vi "Get Header.vi"(8 "error in (no error)":errorcluster, 9 "Default":string, 10 "Header":string, 11 "Request in":refnum<class "Request.lvclass">) -> (0 "error out":errorcluster, 1 "Found?":bool, 2 "Value":string, 3 "Request out":refnum<class "Request.lvclass">)   [LabVIEW 2023, in "Request.lvclass"]
doc: "Returns the value for a given header, if it exists."
uses:
  Request.lvclass
  Request.lvclass/Request.ctl
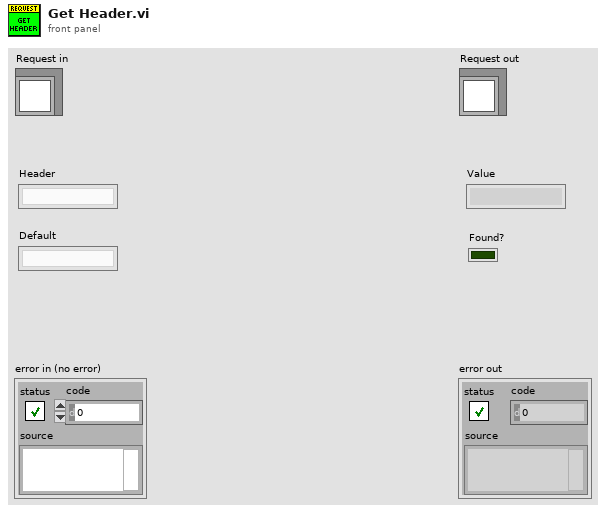
[diagram p1: front panel]
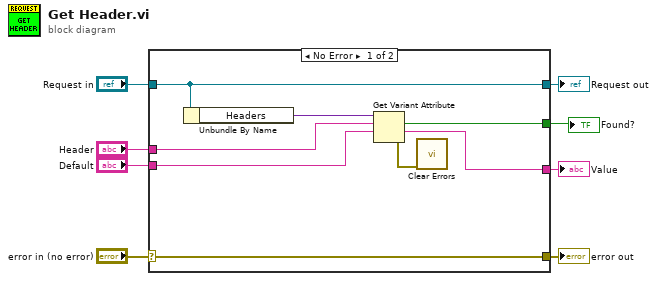
[diagram p0: block diagram]
diagram:
  n1 = case shown="No Error" "error in (no error)" {
    selector: "error in (no error)" -> [w16 w17]
    tunnel: [w16 w17] -> w7
    tunnel: [w15 w18] -> w5
    tunnel: "Request in" -> [w15 w18]
    tunnel: [w11 _] -> w4
    tunnel: "Header" -> [w13 _]
    tunnel: [w10 _] -> w2
    tunnel: "Default" -> [w9 _]
    frame No Error {
      n2 = Unbundle By Name(w15) -> ("Headers"=w14:variant)
      n3 = Get Variant Attribute(Variant=w14, name=w13, default value (empty Variant)=w9) -> (found=w10:bool, value=w11:string, error out=w12:errorcluster)  [unwired: 1 in, 1 out]
      n4 = call <vilib>:"Clear Errors.vi"("error in (no error)"=w12) -> ()  [unwired: 5 in, 2 out]
    }
    frame Error {
    }
  }
  "error out" <- w7
  "Request out" <- w5
  "Value" <- w4
  "Found?" <- w2
